vi "Forward Tell.vi"(8 "Error in":errorcluster, 10 "Msg Attributes":refnum<data-value>, 11 "Base Actor in":refnum<class "Base Actor.lvclass">) -> (0 "Error out":errorcluster, 3 "Base Actor out":refnum<class "Base Actor.lvclass">)   [LabVIEW 2020, in "jettl.lvlib" / "Base jettl Actor.lvlib" / "Base Actor.lvlib" / "Base Actor.lvclass"]
uses:
  Base Actor.lvclass
  Base Actor.lvclass/Base Actor.ctl
  Unified Actor Relation.ctl
  jettl.lvlib
  Msg/Msg.lvclass
  Teller.ctl
  Msg Input/Msg Input.lvclass
  Msg Output/Msg Output.lvclass
  Msg.ctl
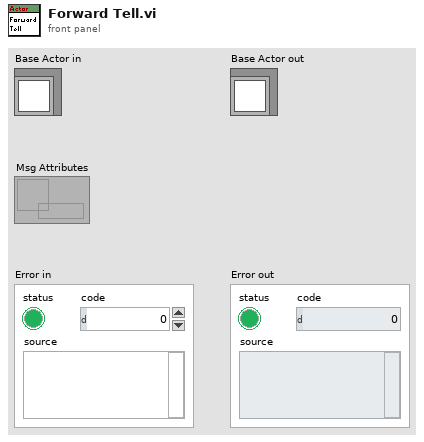
[diagram p1: front panel]
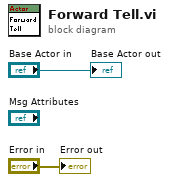
[diagram p0: block diagram]
diagram:
  "Base Actor out" <- "Base Actor in"
  "Error out" <- "Error in"
